vi "Periodic Tasks.vi"(8 "error in":errorcluster) -> ()   [LabVIEW 2015]
doc: "This VI runs in parallel to other tasks. It can contain as many user-defined periodic loops as you need. These can carry out PID or other sorts of timed response."
uses:
  <vilib>/Rock Robotics/WPI/CAN/TalonSRX/WPI_CANTalonSRX_APIControlMode.ctl
  Robot Global Data.vi
  <vilib>/Rock Robotics/Network Tables/NT Write String.vi
  <vilib>/Rock Robotics/WPI/Utilities/WPI_GetSetVariantRefNum.vi
  <vilib>/Rock Robotics/Network Tables/SD Write Numeric Array.vi
  <vilib>/Rock Robotics/Network Tables/SD Write Boolean Array.vi
panel:
  # "PERIODIC TASKS.VI"
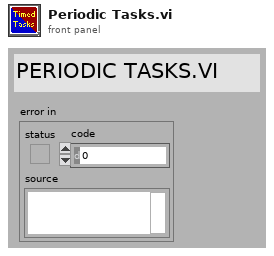
[diagram p1: front panel]
types:
  T1 = typedef "WPI_CANTalonSRX_APIControlMode.ctl" = enum8{"Percent VBus", "Speed", "Position", "Slave", "Unchanged / Invalid", "Voltage Compensation", "Current", "Motion Profile"}
  T2 = typedef "WPI_MotorControlDeviceRef.ctl" = cluster{"DeviceStatus":errorcluster, "Type":T3, "PWM":cluster{"PWM Channel":T4, "DeadBand":T5}, "CAN":cluster{"Device Number":u8, "Control Mode":T6, "Semaphore":T7, "Max Vout":dbl, "TalonSRX Control Mode":T1}, "Invert":bool}
  T3 = typedef "WPI_MotorControlType.ctl" = enum16{"PWM", "CAN", "CANTalonSRX"}
  T4 = typedef "FPGA_DIOPWMChannel.ctl" = enum8{"PWM 0", "PWM 1", "PWM 2", "PWM 3", "PWM 4", "PWM 5", "PWM 6", "PWM 7", "PWM 8", "PWM 9", "PWM MXP 0", "PWM MXP 1", "PWM MXP 2", "PWM MXP 3", "PWM MXP 4", "PWM MXP 5", "PWM MXP 6", "PWM MXP 7", "PWM MXP 8", "PWM MXP 9", "Invalid"}
  T5 = typedef "WPI_PWMDeadband.ctl" = cluster{"Name":string, "maxPositivePwm":i32, "minPositivePwm":i32, "centerPwm":i32, "maxNegativePwm":i32, "minNegativePwm":i32, "angularRange":u16}
  T6 = typedef "WPI_CANJaguar_ControlMode.ctl" = enum8{"Percent VBus", "Current", "Speed", "Position", "Voltage"}
  T7 = typedef "Semaphore RefNum" = refnum<k1>
  T8 = typedef "WPI_JoystickDevRef.ctl" = cluster{"Device":T9}
  T9 = typedef "WPI_JoystickDeviceEnum.ctl" = enum16{"USB 0", "USB 1", "USB 2", "USB 3", "USB 4", "USB 5"}
  T10 = typedef "WPI_ServoDeviceRef.ctl" = cluster{"DeviceStatus":errorcluster, "PWM Channel":T4, "DeadBand":T5}
  T11 = typedef "WPI_PotentiometerDevRef.ctl" = cluster{"DevStatus":errorcluster, "Analog Channel":T12, "Invert Output":bool}
  T12 = typedef "FPGA_AIChannel.ctl" = enum8{"AI 0", "AI 1", "AI 2", "AI 3", "AI MXP 0", "AI MXP 1", "AI MXP 2", "AI MXP 3", "Invalid"}
  T13 = typedef "WPI_SwitchDevRef.ctl" = cluster{"DevStatus":errorcluster, "DIO Channel":T14, "CntIndex":T15, "Normally Closed":bool}
  T14 = typedef "FPGA_DIOChannel.ctl" = enum8{"DIO 0", "DIO 1", "DIO 2", "DIO 3", "DIO 4", "DIO 5", "DIO 6", "DIO 7", "DIO 8", "DIO 9", "DIO MXP 0", "DIO MXP 1", "DIO MXP 2", "DIO MXP 3", "DIO MXP 4", "DIO MXP 5", "DIO MXP 6", "DIO MXP 7", "DIO MXP 8", "DIO MXP 9", "DIO MXP 10", "DIO MXP 11", "DIO MXP 12", "DIO MXP 13", "DIO MXP 14", "DIO MXP 15", "Invalid"}
  T15 = typedef "FPGA_CounterCtrSystemIndex.ctl" = enum8{"Ctr 0", "Ctr 1", "Ctr 2", "Ctr 3", "Ctr 4", "Ctr 5", "Ctr 6", "Ctr 7", "Invalid"}
  T16 = typedef "WPI_CANTalonSRX_GlobalStatus.ctl" = cluster{"Applied Throttle":dbl, "Module Enabled":bool, "CAN Error":errorcluster, "Closed Loop Error":dbl, "Forward Limit Switch Closed":bool, "Reverse Limit Switch Closed":bool, "Sensor Position":dbl, "Sensor Velocity":dbl, "Current":dbl, "Sticky Fault - Over Temp":bool, "Sticky Fault - Under Voltage":bool, "Sticky Fault - Forward Limit":bool, "Sticky Fault - Reverse Limit":bool, "Sticky Fault - Forward Soft Limit":bool, "Sticky Fault - Reverse Soft Limit":bool, "Brake is Enabled":bool, "Encoder Position":dbl, "Encoder Velocity":dbl, "Encoder Index Count":dbl, "Encoder A Pin State":bool, "Encoder B Pin State":bool, "Encoder Index Pin State":bool, "Analog In":dbl, "Analog In Velocity":dbl, "Temperature (C)":dbl, "Battery Voltage":dbl, "Control 5 Is Supported":bool, "Current Profile Slot Select":dbl, "Pos Div 8":bool, "Vel Div 4":bool, "Pulse Width Position":i32, "Pulse Width Velocity":i32, "Pulse Width Rise To Rise (us)":i32, "Pulse Width Rise To Fall (us)":i32, "Mot Prof Active Is Under Run":bool, "Mot Prof Active Has Under Run":bool, "Mot Prof Active Is Last":bool, "Mot Prof Active Velocity Only":bool, "Mot Prof Active Is Valid":bool, "Mot Prof Buffer Is Full":bool, "Mot Prof Active Profile Slot Select":i32, "Mot Prof NextID":i32, "Mot Prof Count":i32, "Mot Prof Active Velocity":dbl, "Mot Prof Active Position":dbl, "Mot Prof Output Enable":i32}
  T17 = typedef "WPI_AnalogChannelDevRef.ctl" = cluster{"DevStatus":errorcluster, "Analog Channel":T12}
  T18 = typedef "WPI_DigitalOutputDevRef.ctl" = cluster{"DIO Channel":T14, "DevStatus":errorcluster}
  T19 = typedef "WPI_GyroDevRef.ctl" = cluster{"DevStatus":errorcluster, "Analog Channel":T12, "Offset":dbl, "Gain (VoltsPerDegree/Second)":dbl, "Gyro Type":enum16{"Analog", "XRS450"}, "Handle":i32, "SPI Bus":T20, "Device Found":bool, "Sample Rate":dbl, "Calibrate On Open":bool}
  T20 = typedef "spi_bus.ctl" = enum16{"SPI On-Board, CS0", "SPI On-Board, CS1", "SPI On-Board, CS2", "SPI On-Board, CS3", "SPI MXP", "Invalid"}
  T21 = typedef "WPI_I2CDevRef.ctl" = cluster{"DevStatus":errorcluster, "Device Address":u8, "Handle":i32, "I2C Bus":T22}
  T22 = typedef "i2c_bus.ctl" = enum16{"I2C On-Board", "I2C MXP", "Invalid"}
  T23 = typedef "WPI_AccelerometerDevRef.ctl" = cluster{"DevStatus":errorcluster, "Scaling":T24, "Analog Channels":T25, "I2C Bus":T22, "SPI Bus":T20, "Accel Range":T26, "ADXL Axes":T27, "Handle":i32, "Device Address":u8, "Accel Type":enum16{"Analog", "ADXL345 I2C", "ADXL345 SPI", "Internal", "ADXL362 SPI"}}
  T24 = typedef "WPI_AccelerometerScaling.ctl" = cluster{"Gain (VoltsPerG)":dbl, "Center Voltage":dbl}
  T25 = typedef "WPI_AccelerometerAnalogChannels.ctl" = cluster{"X-Axis":T12, "Y-Axis":T12, "Z-Axis":T12}
  T26 = typedef "ADXL345 Range.ctl" = u8
  T27 = typedef "WPI_AccelerometerADXL345 Axes.ctl" = cluster{"X-Axis":bool, "Y-Axis":bool, "Z-Axis":bool}
  T28 = cluster{"X-Axis":dbl, "Y-Axis":dbl, "Z-Axis":dbl}
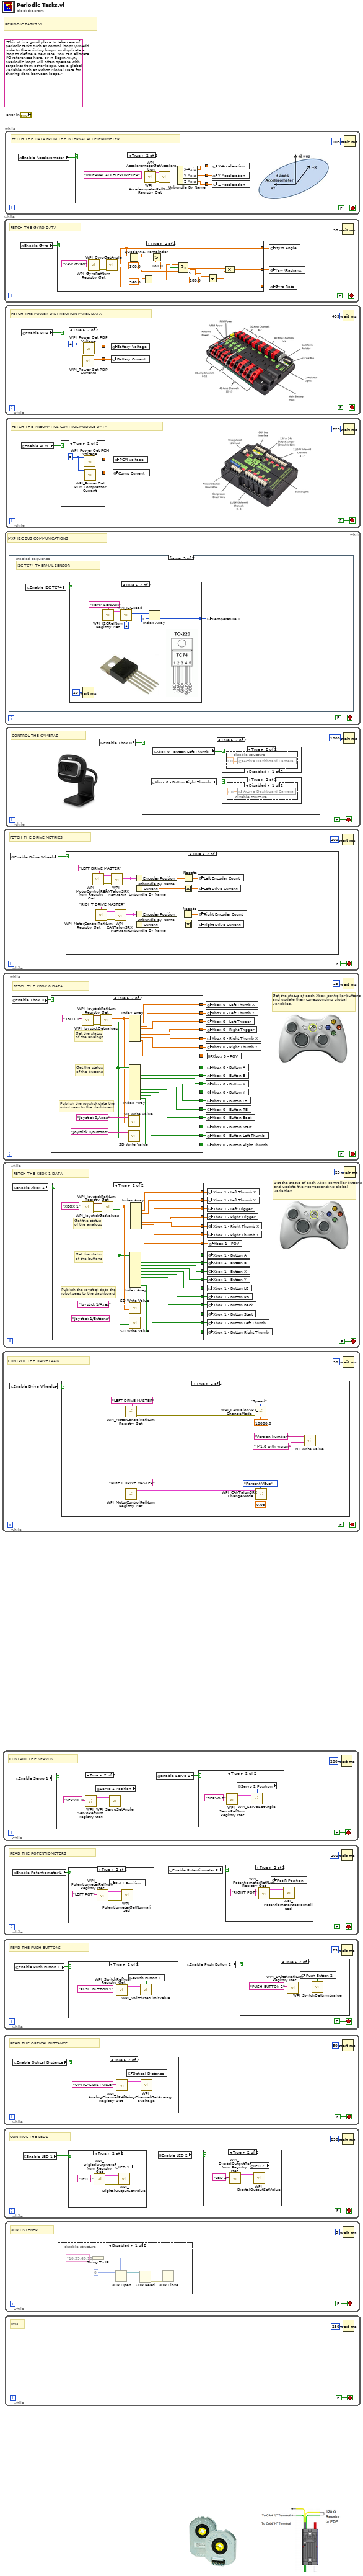
[diagram p0: block diagram]
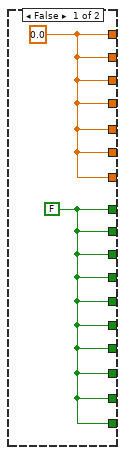
[diagram p12: hidden frame]
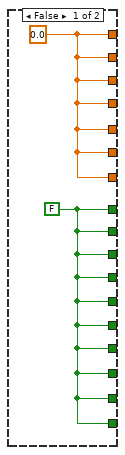
[diagram p13: hidden frame]
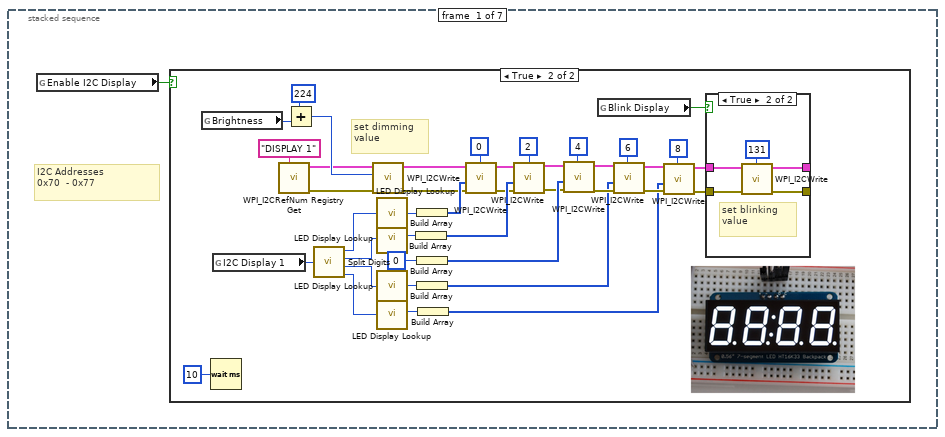
[diagram p14: hidden frame]
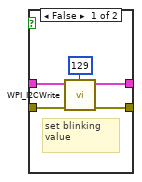
[diagram p16: hidden frame]
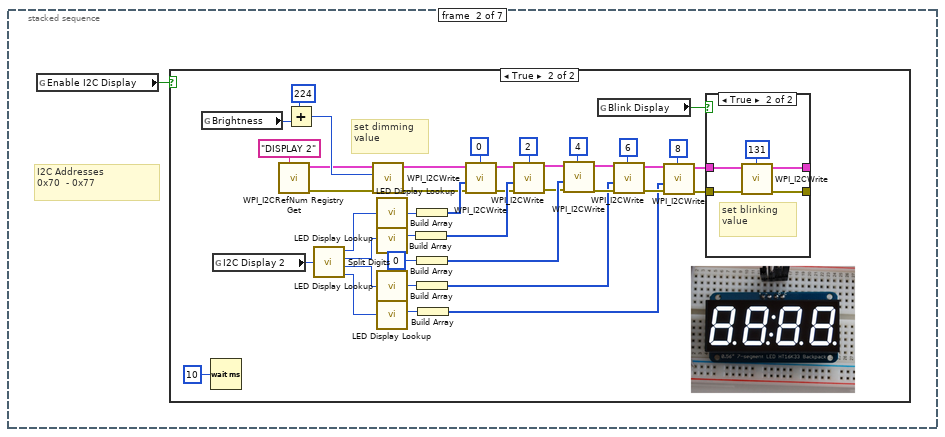
[diagram p17: hidden frame]
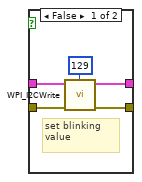
[diagram p19: hidden frame]
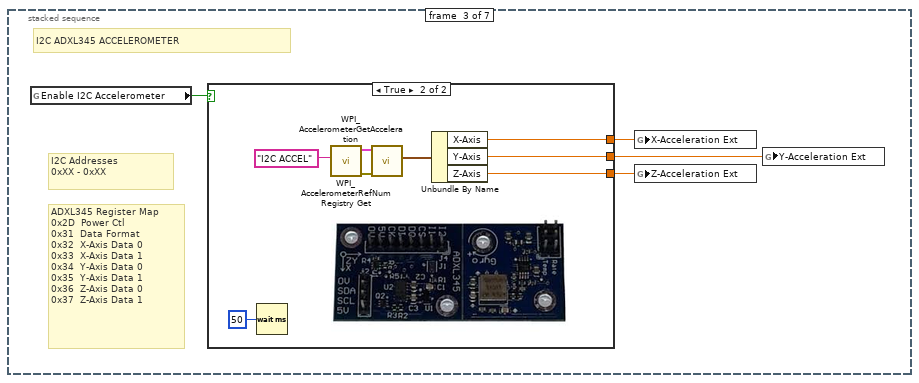
[diagram p20: hidden frame]
diagram:
  (unwired) "This VI is a good place to take care of periodic tasks such as control loops.\n\nAdd code to the existing loops, or duplicate a loop to define a new rate. You can allocate I/O references here, or in Begin.vi.\n\nPeriodic loops will often operate with setpoints from other loops. Use a global variable such as Robot Global Data for sharing data between loops."
  # "PERIODIC TASKS.VI"
  n1 = while {
    stop <- FALSE stop-if-true
    # "CONTROL THE DRIVETRAIN"
    n2 = global read "Robot Global Data.vi" "Enable Drive Wheels"() -> (w1:bool)
    n3 = case shown="True" w1 {
      frame False {
      }
      frame True {
        n4 = call <vilib>:"WPI_MotorControlRefNum Registry Get.vi"("refnum name"="LEFT DRIVE MASTER") -> ("error out"=w13:errorcluster, "MotorControlDevRef"=w14:T2)  [unwired: 9 in]
        n5 = call <vilib>:"WPI_MotorControlRefNum Registry Get.vi"("refnum name"="RIGHT DRIVE MASTER") -> ("error out"=w4:errorcluster, "MotorControlDevRef"=w5:T2)  [unwired: 9 in]
        n6 = call <vilib>:"WPI_CANTalonSRX_ChangeMode.vi"("error in (no error)"=w13, "Output"=10000.0, "Control Mode"=WPI_CANTalonSRX_APIControlMode."Speed", "CAN Talon SRX Ref"=w14) -> ()  [unwired: 6 in, 2 out]
        n7 = call <vilib>:"WPI_CANTalonSRX_ChangeMode.vi"("error in (no error)"=w4, "Output"=0.09, "Control Mode"=WPI_CANTalonSRX_APIControlMode."Percent VBus", "CAN Talon SRX Ref"=w5) -> ()  [unwired: 6 in, 2 out]
        n8 = call-poly <vilib>:"NT Write Value.vi"("String"=" M1.0 with vision", "Name"="Version Number") -> ()  [unwired: 9 in, 1 out]
      }
    }
    n9 = Wait (ms)(milliseconds to wait=u32 50) -> ()  [unwired: 1 out]
  }
  n10 = while {
    stop <- FALSE stop-if-true
    # "Get the status of each Xbox controller buttons and update their corresponding global variables."
    # "FETCH THE XBOX 0 DATA"
    n11 = global read "Robot Global Data.vi" "Enable Xbox 0"() -> (w35:bool)
    n12 = case shown="True" w35 {
      tunnel: [w36 w61] -> w34
      tunnel: [w36 w60] -> w33
      tunnel: [w36 w59] -> w32
      tunnel: [w37 w58] -> w31
      tunnel: [w37 w57] -> w30
      tunnel: [w37 w56] -> w29
      tunnel: [w37 w55] -> w28
      tunnel: [w37 w54] -> w27
      tunnel: [w37 w53] -> w26
      tunnel: [w37 w52] -> w25
      tunnel: [w37 w51] -> w24
      tunnel: [w37 w50] -> w23
      tunnel: [w37 w49] -> w22
      tunnel: [w36 w48] -> w21
      tunnel: [w36 w47] -> w20
      tunnel: [w36 w46] -> w19
      tunnel: [w36 w45] -> w18
      frame False {
        w36 = 0.0 ("upper limit")
        w37 = FALSE
      }
      frame True {
        # "Publish the joystick data the\nrobot sees to the dashboard"
        # "Get the status\nof the analogs"
        # "Get the status\nof the buttons"
        n13 = call <vilib>:"WPI_JoystickRefNum Registry Get.vi"("refnum name"="XBOX 0") -> ("error out"=w38:errorcluster, "JoystickDevRef"=w39:T8)  [unwired: 9 in]
        n14 = call <vilib>:"WPI_JoystickGetValues.vi"("error in (no error)"=w38, "JoystickDevRef"=w39) -> ("Buttons"=w42:bool[], "Axes"=w41:dbl[])  [unwired: 5 in, 3 out]
        n15 = call-poly <vilib>:"SD Write Value.vi"("Numeric Array"=w41, "Name"="Joystick 0/Axes") -> ()  [unwired: 8 in, 2 out]
        n16 = call-poly <vilib>:"SD Write Value.vi"("Boolean Array"=w42, "Name"="Joystick 0/Buttons") -> ()  [unwired: 8 in, 2 out]
        n17 = Index Array(array=w42) -> (element #1=w58:bool, element #2=w57:bool, element #3=w56:bool, element #4=w55:bool, element #5=w54:bool, element #6=w53:bool, element #7=w52:bool, element #8=w51:bool, element #9=w50:bool, element #10=w49:bool)  [unwired: 10 in]
        n18 = Index Array(array=w41) -> (element #1=w61:dbl, element #2=w60:dbl, element #3=w59:dbl, element #4=w48:dbl, element #5=w47:dbl, element #6=w46:dbl, element #7=w45:dbl)  [unwired: 7 in]
      }
    }
    n19 = global write "Robot Global Data.vi" "Xbox 0 - Left Thumb X"(w34) -> ()
    n20 = global write "Robot Global Data.vi" "Xbox 0 - Left Thumb Y"(w33) -> ()
    n21 = global write "Robot Global Data.vi" "Xbox 0 - Left Trigger"(w32) -> ()
    n22 = global write "Robot Global Data.vi" "Xbox 0 - Right Trigger"(w21) -> ()
    n23 = global write "Robot Global Data.vi" "Xbox 0 - Right Thumb X"(w20) -> ()
    n24 = global write "Robot Global Data.vi" "Xbox 0 - Right Thumb Y"(w19) -> ()
    n25 = global write "Robot Global Data.vi" "Xbox 0 - Button A"(w31) -> ()
    n26 = global write "Robot Global Data.vi" "Xbox 0 - Button B"(w30) -> ()
    n27 = global write "Robot Global Data.vi" "Xbox 0 - Button X"(w29) -> ()
    n28 = global write "Robot Global Data.vi" "Xbox 0 - Button Y"(w28) -> ()
    n29 = global write "Robot Global Data.vi" "Xbox 0 - Button LB"(w27) -> ()
    n30 = global write "Robot Global Data.vi" "Xbox 0 - Button RB"(w26) -> ()
    n31 = global write "Robot Global Data.vi" "Xbox 0 - Button Back"(w25) -> ()
    n32 = global write "Robot Global Data.vi" "Xbox 0 - Button Start"(w24) -> ()
    n33 = global write "Robot Global Data.vi" "Xbox 0 - Button Left Thumb"(w23) -> ()
    n34 = global write "Robot Global Data.vi" "Xbox 0 - Button Right Thumb"(w22) -> ()
    n35 = global write "Robot Global Data.vi" "Xbox 0 - POV"(w18) -> ()
    n36 = Wait (ms)(milliseconds to wait=u32 25) -> ()  [unwired: 1 out]
  }
  n37 = while {
    stop <- FALSE stop-if-true
    # "Get the status of each Xbox controller buttons and update their corresponding global variables."
    # "FETCH THE XBOX 1 DATA"
    n38 = global read "Robot Global Data.vi" "Enable Xbox 1"() -> (w81:bool)
    n39 = case shown="True" w81 {
      tunnel: [w82 w107] -> w80
      tunnel: [w82 w106] -> w79
      tunnel: [w82 w105] -> w78
      tunnel: [w83 w104] -> w77
      tunnel: [w83 w103] -> w76
      tunnel: [w83 w102] -> w75
      tunnel: [w83 w101] -> w74
      tunnel: [w83 w100] -> w73
      tunnel: [w83 w99] -> w72
      tunnel: [w83 w98] -> w71
      tunnel: [w83 w97] -> w70
      tunnel: [w83 w96] -> w69
      tunnel: [w83 w95] -> w68
      tunnel: [w82 w94] -> w67
      tunnel: [w82 w93] -> w66
      tunnel: [w82 w92] -> w65
      tunnel: [w82 w91] -> w64
      frame False {
        w82 = 0.0 ("upper limit")
        w83 = FALSE
      }
      frame True {
        # "Publish the joystick data the\nrobot sees to the dashboard"
        # "Get the status\nof the analogs"
        # "Get the status\nof the buttons"
        n40 = call <vilib>:"WPI_JoystickRefNum Registry Get.vi"("refnum name"="XBOX 1") -> ("error out"=w84:errorcluster, "JoystickDevRef"=w85:T8)  [unwired: 9 in]
        n41 = call <vilib>:"WPI_JoystickGetValues.vi"("error in (no error)"=w84, "JoystickDevRef"=w85) -> ("Buttons"=w87:bool[], "Axes"=w88:dbl[])  [unwired: 5 in, 3 out]
        n42 = call-poly <vilib>:"SD Write Value.vi"("Numeric Array"=w88, "Name"="Joystick 1/Axes") -> ()  [unwired: 8 in, 2 out]
        n43 = call-poly <vilib>:"SD Write Value.vi"("Boolean Array"=w87, "Name"="Joystick 1/Buttons") -> ()  [unwired: 8 in, 2 out]
        n44 = Index Array(array=w87) -> (element #1=w104:bool, element #2=w103:bool, element #3=w102:bool, element #4=w101:bool, element #5=w100:bool, element #6=w99:bool, element #7=w98:bool, element #8=w97:bool, element #9=w96:bool, element #10=w95:bool)  [unwired: 10 in]
        n45 = Index Array(array=w88) -> (element #1=w107:dbl, element #2=w106:dbl, element #3=w105:dbl, element #4=w94:dbl, element #5=w93:dbl, element #6=w92:dbl, element #7=w91:dbl)  [unwired: 7 in]
      }
    }
    n46 = global write "Robot Global Data.vi" "Xbox 1 - Left Thumb X"(w80) -> ()
    n47 = global write "Robot Global Data.vi" "Xbox 1 - Left Thumb Y"(w79) -> ()
    n48 = global write "Robot Global Data.vi" "Xbox 1 - Left Trigger"(w78) -> ()
    n49 = global write "Robot Global Data.vi" "Xbox 1 - Right Trigger"(w67) -> ()
    n50 = global write "Robot Global Data.vi" "Xbox 1 - Right Thumb X"(w66) -> ()
    n51 = global write "Robot Global Data.vi" "Xbox 1 - Right Thumb Y"(w65) -> ()
    n52 = global write "Robot Global Data.vi" "Xbox 1 - Button A"(w77) -> ()
    n53 = global write "Robot Global Data.vi" "Xbox 1 - Button B"(w76) -> ()
    n54 = global write "Robot Global Data.vi" "Xbox 1 - Button X"(w75) -> ()
    n55 = global write "Robot Global Data.vi" "Xbox 1 - Button Y"(w74) -> ()
    n56 = global write "Robot Global Data.vi" "Xbox 1 - Button LB"(w73) -> ()
    n57 = global write "Robot Global Data.vi" "Xbox 1 - Button RB"(w72) -> ()
    n58 = global write "Robot Global Data.vi" "Xbox 1 - Button Back"(w71) -> ()
    n59 = global write "Robot Global Data.vi" "Xbox 1 - Button Start"(w70) -> ()
    n60 = global write "Robot Global Data.vi" "Xbox 1 - Button Left Thumb"(w69) -> ()
    n61 = global write "Robot Global Data.vi" "Xbox 1 - Button Right Thumb"(w68) -> ()
    n62 = global write "Robot Global Data.vi" "Xbox 1 - POV"(w64) -> ()
    n63 = Wait (ms)(milliseconds to wait=u32 25) -> ()  [unwired: 1 out]
  }
  n64 = while {
    stop <- FALSE stop-if-true
    # "CONTROL THE SERVOS"
    n65 = global read "Robot Global Data.vi" "Enable Servo 1"() -> (w109:bool)
    n66 = case shown="True" w109 {
      frame False {
      }
      frame True {
        n67 = call <vilib>:"WPI_ServoRefNum Registry Get.vi"("refnum name"="SERVO 1") -> ("error out"=w118:errorcluster, "ServoDeviceRef"=w117:T10)  [unwired: 9 in]
        n68 = global read "Robot Global Data.vi" "Servo 1 Position"() -> (w116:i32)
        n69 = call <vilib>:"WPI_ServoSetAngle.vi"("error in (no error)"=w118, "Angle"=w116, "ServoDeviceRef"=w117) -> ()  [unwired: 7 in, 2 out]
      }
    }
    n70 = global read "Robot Global Data.vi" "Enable Servo 1"() -> (w108:bool)
    n71 = case shown="True" w108 {
      frame False {
      }
      frame True {
        n72 = call <vilib>:"WPI_ServoRefNum Registry Get.vi"("refnum name"="SERVO 2") -> ("error out"=w114:errorcluster, "ServoDeviceRef"=w113:T10)  [unwired: 9 in]
        n73 = global read "Robot Global Data.vi" "Servo 2 Position"() -> (w112:i32)
        n74 = call <vilib>:"WPI_ServoSetAngle.vi"("error in (no error)"=w114, "Angle"=w112, "ServoDeviceRef"=w113) -> ()  [unwired: 7 in, 2 out]
      }
    }
    n75 = Wait (ms)(milliseconds to wait=u32 200) -> ()  [unwired: 1 out]
  }
  n76 = while {
    stop <- FALSE stop-if-true
    # "READ THE POTENTIOMETERS"
    n77 = global read "Robot Global Data.vi" "Enable Potentiometer L"() -> (w121:bool)
    n78 = case shown="True" w121 {
      frame False {
      }
      frame True {
        n79 = call <vilib>:"WPI_PotentiometerRefNum Registry Get.vi"("refnum name"="LEFT POT") -> ("error out"=w130:errorcluster, "PotDevRef"=w129:T11)  [unwired: 9 in]
        n80 = call <vilib>:"WPI_PotentiometerGetNormalized.vi"("error in"=w130, "PotDevRef"=w129) -> ("Normalized Value"=w128:dbl)  [unwired: 7 in, 2 out]
        n81 = global write "Robot Global Data.vi" "Pot L Position"(w128) -> ()
      }
    }
    n82 = global read "Robot Global Data.vi" "Enable Potentiometer R"() -> (w120:bool)
    n83 = case shown="True" w120 {
      frame False {
      }
      frame True {
        n84 = call <vilib>:"WPI_PotentiometerRefNum Registry Get.vi"("refnum name"="RIGHT POT") -> ("error out"=w126:errorcluster, "PotDevRef"=w125:T11)  [unwired: 9 in]
        n85 = call <vilib>:"WPI_PotentiometerGetNormalized.vi"("error in"=w126, "PotDevRef"=w125) -> ("Normalized Value"=w124:dbl)  [unwired: 7 in, 2 out]
        n86 = global write "Robot Global Data.vi" "Pot R Position"(w124) -> ()
      }
    }
    n87 = Wait (ms)(milliseconds to wait=u32 200) -> ()  [unwired: 1 out]
  }
  n88 = while {
    stop <- FALSE stop-if-true
    # "READ THE PUSH BUTTONS"
    n89 = global read "Robot Global Data.vi" "Enable Push Button 1"() -> (w133:bool)
    n90 = case shown="True" w133 {
      frame False {
      }
      frame True {
        n91 = call <vilib>:"WPI_SwitchRefNum Registry Get.vi"("refnum name"="PUSH BUTTON 1") -> ("error out"=w142:errorcluster, "SwitchDevRef"=w141:T13)  [unwired: 9 in]
        n92 = call <vilib>:"WPI_SwitchGetLimitValue.vi"("error in (no error)"=w142, "SwitchDevRef"=w141) -> ("Switch Pressed"=w140:bool)  [unwired: 7 in, 2 out]
        n93 = global write "Robot Global Data.vi" "Push Button 1"(w140) -> ()
      }
    }
    n94 = global read "Robot Global Data.vi" "Enable Push Button 2"() -> (w132:bool)
    n95 = case shown="True" w132 {
      frame False {
      }
      frame True {
        n96 = call <vilib>:"WPI_SwitchRefNum Registry Get.vi"("refnum name"="PUSH BUTTON 2") -> ("error out"=w138:errorcluster, "SwitchDevRef"=w137:T13)  [unwired: 9 in]
        n97 = call <vilib>:"WPI_SwitchGetLimitValue.vi"("error in (no error)"=w138, "SwitchDevRef"=w137) -> ("Switch Pressed"=w136:bool)  [unwired: 7 in, 2 out]
        n98 = global write "Robot Global Data.vi" "Push Button 2"(w136) -> ()
      }
    }
    n99 = Wait (ms)(milliseconds to wait=u32 25) -> ()  [unwired: 1 out]
  }
  n100 = while {
    stop <- FALSE stop-if-true
    # "FETCH THE DRIVE METRICS"
    n101 = global read "Robot Global Data.vi" "Enable Drive Wheels"() -> (w144:bool)
    n102 = case shown="True" w144 {
      frame False {
      }
      frame True {
        n103 = call <vilib>:"WPI_MotorControlRefNum Registry Get.vi"("refnum name"="LEFT DRIVE MASTER") -> ("error out"=w160:errorcluster, "MotorControlDevRef"=w161:T2)  [unwired: 9 in]
        n104 = call <vilib>:"WPI_MotorControlRefNum Registry Get.vi"("refnum name"="RIGHT DRIVE MASTER") -> ("error out"=w157:errorcluster, "MotorControlDevRef"=w158:T2)  [unwired: 9 in]
        n105 = call <vilib>:"WPI_CANTalonSRX_GetStatus.vi"("error in (no error)"=w160, "CAN Talon SRX Ref"=w161) -> ("Talon SRX Status"=w151:T16)  [unwired: 7 in, 2 out]
        n106 = call <vilib>:"WPI_CANTalonSRX_GetStatus.vi"("error in (no error)"=w157, "CAN Talon SRX Ref"=w158) -> ("Talon SRX Status"=w156:T16)  [unwired: 7 in, 2 out]
        n107 = Unbundle By Name(w151) -> ("Encoder Position"=w149:dbl)
        n108 = Unbundle By Name(w151) -> ("Current"=w153:dbl)
        n109 = Unbundle By Name(w156) -> ("Encoder Position"=w148:dbl)
        n110 = Unbundle By Name(w156) -> ("Current"=w155:dbl)
        n111 = Negate(x=w148) -> (-x=w147:dbl)
        n112 = Absolute Value(x=w153) -> (abs(x)=w152:dbl)
        n113 = Absolute Value(x=w155) -> (abs(x)=w154:dbl)
        n114 = Negate(x=w149) -> (-x=w150:dbl)
        n115 = global write "Robot Global Data.vi" "Left Encoder Count"(w150) -> ()
        n116 = global write "Robot Global Data.vi" "Left Drive Current"(w152) -> ()
        n117 = global write "Robot Global Data.vi" "Right Encoder Count"(w147) -> ()
        n118 = global write "Robot Global Data.vi" "Right Drive Current"(w154) -> ()
      }
    }
    n119 = Wait (ms)(milliseconds to wait=u32 200) -> ()  [unwired: 1 out]
  }
  n120 = while {
    stop <- FALSE stop-if-true
    # "READ THE OPTICAL DISTANCE"
    n121 = global read "Robot Global Data.vi" "Enable Optical Distance"() -> (w163:bool)
    n122 = case shown="True" w163 {
      frame False {
      }
      frame True {
        n123 = call <vilib>:"WPI_AnalogChannelRefNum Registry Get.vi"("refnum name"="OPTICAL DISTANCE") -> ("error out"=w168:errorcluster, "AIDeviceRef"=w167:T17)  [unwired: 9 in]
        n124 = call <vilib>:"WPI_AnalogChannelGetAverageVoltage.vi"("error in (no error)"=w168, "AIDeviceRef"=w167) -> ("Voltage"=w166:dbl)  [unwired: 7 in, 2 out]
        n125 = global write "Robot Global Data.vi" "Optical Distance"(w166) -> ()
      }
    }
    n126 = Wait (ms)(milliseconds to wait=u32 50) -> ()  [unwired: 1 out]
  }
  n127 = while {
    stop <- FALSE stop-if-true
    # "CONTROL THE LEDS"
    n128 = global read "Robot Global Data.vi" "Enable LED 1"() -> (w171:bool)
    n129 = case shown="True" w171 {
      frame False {
      }
      frame True {
        n130 = call <vilib>:"WPI_DigitalOutputRefNum Registry Get.vi"("refnum name"="LED 1") -> ("error out"=w180:errorcluster, "DigitalOutputDevRef"=w179:T18)  [unwired: 9 in]
        n131 = global read "Robot Global Data.vi" "LED 1"() -> (w178:bool)
        n132 = call <vilib>:"WPI_DigitalOutputSetValue.vi"("error in (no error)"=w180, "Value"=w178, "DigitalOutputDevRef"=w179) -> ()  [unwired: 7 in, 2 out]
      }
    }
    n133 = global read "Robot Global Data.vi" "Enable LED 2"() -> (w170:bool)
    n134 = case shown="True" w170 {
      frame False {
      }
      frame True {
        n135 = call <vilib>:"WPI_DigitalOutputRefNum Registry Get.vi"("refnum name"="LED 2") -> ("error out"=w176:errorcluster, "DigitalOutputDevRef"=w175:T18)  [unwired: 9 in]
        n136 = global read "Robot Global Data.vi" "LED 2"() -> (w174:bool)
        n137 = call <vilib>:"WPI_DigitalOutputSetValue.vi"("error in (no error)"=w176, "Value"=w174, "DigitalOutputDevRef"=w175) -> ()  [unwired: 7 in, 2 out]
      }
    }
    n138 = Wait (ms)(milliseconds to wait=u32 250) -> ()  [unwired: 1 out]
  }
  n139 = while {
    stop <- FALSE stop-if-true
    # "FETCH THE GYRO DATA"
    n140 = global read "Robot Global Data.vi" "Enable Gyro"() -> (w185:bool)
    n141 = case shown="True" w185 {
      tunnel: [w188 w200] -> w183
      tunnel: [w188 w204] -> w184
      tunnel: [w188 w189] -> w182
      frame False {
        w188 = 0.0
      }
      frame True {
        n142 = call <vilib>:"WPI_GyroRefNum Registry Get.vi"("refnum name"="YAW GYRO") -> ("error out"=w201:errorcluster, "GyroDevRef"=w202:T19)  [unwired: 9 in]
        n143 = call <vilib>:"WPI_GyroGetAngle.vi"("error in"=w201, "GyroDevRef"=w202) -> ("Angular Rate"=w204:dbl, "Angle"=w200:dbl)  [unwired: 5 in, 3 out]
        n144 = Quotient & Remainder(x=w200, y=360.0) -> (x-y*floor(x/y)=w194:dbl)  [unwired: 1 out]
        n145 = Subtract(x=w194, y=360.0) -> (x-y=w195:dbl)
        n146 = Greater?(x=w194, y=180.0) -> (0:w196:bool)
        n147 = Select(t=w195, s=w196, f=w194) -> (s? t:f=w191:dbl)
        n148 = Divide(x=3.141592653589793, y=180.0) -> (x/y=w190:dbl)
        n149 = Compound Arithmetic op=MULTIPLY(w191, w190) -> (w189:dbl)
      }
    }
    n150 = global write "Robot Global Data.vi" "Gyro Angle"(w183) -> ()
    n151 = global write "Robot Global Data.vi" "Yaw (Radians)"(w182) -> ()
    n152 = global write "Robot Global Data.vi" "Gyro Rate"(w184) -> ()
    n153 = Wait (ms)(milliseconds to wait=u32 97) -> ()  [unwired: 1 out]
  }
  n154 = while {
    stop <- FALSE stop-if-true
    # "MXP I2C BUS COMMUNICATIONS"
    n155 = stacked-sequence {
      frame #0 {
        # "I2C Addresses\n0x70  - 0x77"
        n156 = global read "Robot Global Data.vi" "Enable I2C Display"() -> (w206:bool)
        n157 = case shown="True" w206 {
          frame False {
          }
          frame True {
            # "set dimming value"
            n158 = global read "Robot Global Data.vi" "Brightness"() -> (w223:u8)
            n159 = Wait (ms)(milliseconds to wait=u32 10) -> ()  [unwired: 1 out]
            n160 = global read "Robot Global Data.vi" "I2C Display 1"() -> (w221:u16)
            n161 = call <vilib>:"WPI_I2CRefNum Registry Get.vi"("refnum name"="DISPLAY 1") -> ("error out"=w208:errorcluster, "I2CDevRef"=w209:T21)  [unwired: 9 in]
            n162 = Add(x=u8 224 ("I2CRegister"), y=w223) -> (x+y=w222:u8)
            n163 = call "Split Digits.vi"("Input"=w221) -> ("Digit 4"=w213:u16, "Digit 3"=w214:u16, "Digit 2"=w215:u16, "Digit 1"=w216:u16)
            n164 = call <vilib>:"WPI_I2CWrite.vi"("error in (no error)"=w208, "I2CRegister"=w222, "I2CDevRef"=w209) -> ("error out"=w211:errorcluster, "I2CDevRef"=w212:T21)  [unwired: 7 in]
            n165 = call "LED Display Lookup.vi"("Input"=w213) -> ("Output"=w228:u8)
            n166 = call "LED Display Lookup.vi"("Input"=w214) -> ("Output"=w218:u8)
            n167 = call "LED Display Lookup.vi"("Input"=w215) -> ("Output"=w219:u8)
            n168 = call "LED Display Lookup.vi"("Input"=w216) -> ("Output"=w220:u8)
            n169 = Build Array(w218) -> (w243:u8[])
            n170 = Build Array(w228) -> (w245:u8[])
            n171 = Build Array(u8 0 ("Data To Send")) -> (w239:u8[])
            n172 = Build Array(w219) -> (w232:u8[])
            n173 = Build Array(w220) -> (w229:u8[])
            n174 = call <vilib>:"WPI_I2CWrite.vi"("error in (no error)"=w211, "I2CDataToSend"=w245, "I2CRegister"=u8 0 ("Data To Send"), "I2CDevRef"=w212) -> ("error out"=w241:errorcluster, "I2CDevRef"=w242:T21)  [unwired: 6 in]
            n175 = call <vilib>:"WPI_I2CWrite.vi"("error in (no error)"=w241, "I2CDataToSend"=w243, "I2CRegister"=u8 2 ("Data To Send"), "I2CDevRef"=w242) -> ("error out"=w237:errorcluster, "I2CDevRef"=w238:T21)  [unwired: 6 in]
            n176 = call <vilib>:"WPI_I2CWrite.vi"("error in (no error)"=w237, "I2CDataToSend"=w239, "I2CRegister"=u8 4 ("Data To Send"), "I2CDevRef"=w238) -> ("error out"=w233:errorcluster, "I2CDevRef"=w234:T21)  [unwired: 6 in]
            n177 = global read "Robot Global Data.vi" "Blink Display"() -> (w225:bool)
            n178 = call <vilib>:"WPI_I2CWrite.vi"("error in (no error)"=w233, "I2CDataToSend"=w232, "I2CRegister"=u8 6 ("Data To Send"), "I2CDevRef"=w234) -> ("error out"=w230:errorcluster, "I2CDevRef"=w231:T21)  [unwired: 6 in]
            n179 = call <vilib>:"WPI_I2CWrite.vi"("error in (no error)"=w230, "I2CDataToSend"=w229, "I2CRegister"=u8 8 ("Data To Send"), "I2CDevRef"=w231) -> ("error out"=w226:errorcluster, "I2CDevRef"=w227:T21)  [unwired: 6 in]
            n180 = case shown="True" w225 {
              tunnel: [w248 w255] -> _
              tunnel: [w247 w254] -> _
              tunnel: w227 -> [w250 w253]
              tunnel: w226 -> [w249 w252]
              frame False {
                # "set blinking value"
                n181 = call <vilib>:"WPI_I2CWrite.vi"("error in (no error)"=w249, "I2CRegister"=u8 129, "I2CDevRef"=w250) -> ("error out"=w247:errorcluster, "I2CDevRef"=w248:T21)  [unwired: 7 in]
              }
              frame True {
                # "set blinking value"
                n182 = call <vilib>:"WPI_I2CWrite.vi"("error in (no error)"=w252, "I2CRegister"=u8 131, "I2CDevRef"=w253) -> ("error out"=w254:errorcluster, "I2CDevRef"=w255:T21)  [unwired: 7 in]
              }
            }
          }
        }
      }
      frame #1 {
        # "I2C Addresses\n0x70  - 0x77"
        n183 = global read "Robot Global Data.vi" "Enable I2C Display"() -> (w257:bool)
        n184 = case shown="True" w257 {
          frame False {
          }
          frame True {
            # "set dimming value"
            n185 = global read "Robot Global Data.vi" "Brightness"() -> (w274:u8)
            n186 = Wait (ms)(milliseconds to wait=u32 10) -> ()  [unwired: 1 out]
            n187 = global read "Robot Global Data.vi" "I2C Display 2"() -> (w272:u16)
            n188 = call <vilib>:"WPI_I2CRefNum Registry Get.vi"("refnum name"="DISPLAY 2") -> ("error out"=w259:errorcluster, "I2CDevRef"=w260:T21)  [unwired: 9 in]
            n189 = Add(x=u8 224 ("I2CRegister"), y=w274) -> (x+y=w273:u8)
            n190 = call "Split Digits.vi"("Input"=w272) -> ("Digit 4"=w264:u16, "Digit 3"=w265:u16, "Digit 2"=w266:u16, "Digit 1"=w267:u16)
            n191 = call <vilib>:"WPI_I2CWrite.vi"("error in (no error)"=w259, "I2CRegister"=w273, "I2CDevRef"=w260) -> ("error out"=w262:errorcluster, "I2CDevRef"=w263:T21)  [unwired: 7 in]
            n192 = call "LED Display Lookup.vi"("Input"=w264) -> ("Output"=w279:u8)
            n193 = call "LED Display Lookup.vi"("Input"=w265) -> ("Output"=w269:u8)
            n194 = call "LED Display Lookup.vi"("Input"=w266) -> ("Output"=w270:u8)
            n195 = call "LED Display Lookup.vi"("Input"=w267) -> ("Output"=w271:u8)
            n196 = Build Array(w269) -> (w294:u8[])
            n197 = Build Array(w279) -> (w296:u8[])
            n198 = Build Array(u8 0 ("Data To Send")) -> (w290:u8[])
            n199 = Build Array(w270) -> (w283:u8[])
            n200 = Build Array(w271) -> (w280:u8[])
            n201 = call <vilib>:"WPI_I2CWrite.vi"("error in (no error)"=w262, "I2CDataToSend"=w296, "I2CRegister"=u8 0 ("Data To Send"), "I2CDevRef"=w263) -> ("error out"=w292:errorcluster, "I2CDevRef"=w293:T21)  [unwired: 6 in]
            n202 = call <vilib>:"WPI_I2CWrite.vi"("error in (no error)"=w292, "I2CDataToSend"=w294, "I2CRegister"=u8 2 ("Data To Send"), "I2CDevRef"=w293) -> ("error out"=w288:errorcluster, "I2CDevRef"=w289:T21)  [unwired: 6 in]
            n203 = call <vilib>:"WPI_I2CWrite.vi"("error in (no error)"=w288, "I2CDataToSend"=w290, "I2CRegister"=u8 4 ("Data To Send"), "I2CDevRef"=w289) -> ("error out"=w284:errorcluster, "I2CDevRef"=w285:T21)  [unwired: 6 in]
            n204 = global read "Robot Global Data.vi" "Blink Display"() -> (w276:bool)
            n205 = call <vilib>:"WPI_I2CWrite.vi"("error in (no error)"=w284, "I2CDataToSend"=w283, "I2CRegister"=u8 6 ("Data To Send"), "I2CDevRef"=w285) -> ("error out"=w281:errorcluster, "I2CDevRef"=w282:T21)  [unwired: 6 in]
            n206 = call <vilib>:"WPI_I2CWrite.vi"("error in (no error)"=w281, "I2CDataToSend"=w280, "I2CRegister"=u8 8 ("Data To Send"), "I2CDevRef"=w282) -> ("error out"=w277:errorcluster, "I2CDevRef"=w278:T21)  [unwired: 6 in]
            n207 = case shown="True" w276 {
              tunnel: [w299 w306] -> _
              tunnel: [w298 w305] -> _
              tunnel: w278 -> [w301 w304]
              tunnel: w277 -> [w300 w303]
              frame False {
                # "set blinking value"
                n208 = call <vilib>:"WPI_I2CWrite.vi"("error in (no error)"=w300, "I2CRegister"=u8 129, "I2CDevRef"=w301) -> ("error out"=w298:errorcluster, "I2CDevRef"=w299:T21)  [unwired: 7 in]
              }
              frame True {
                # "set blinking value"
                n209 = call <vilib>:"WPI_I2CWrite.vi"("error in (no error)"=w303, "I2CRegister"=u8 131, "I2CDevRef"=w304) -> ("error out"=w305:errorcluster, "I2CDevRef"=w306:T21)  [unwired: 7 in]
              }
            }
          }
        }
      }
      frame #2 {
        # "I2C Addresses\n0xXX - 0xXX"
        # "ADXL345 Register Map\n0x2D  Power Ctl\n0x31  Data Format\n0x32  X-Axis Data 0\n0x33  X-Axis Data 1\n0x34  Y-Axis Data 0\n0x35  Y-Axis Data 1\n0x36  Z-Axis Data 0\n0x37  Z-Axis Data 1"
        # "I2C ADXL345 ACCELEROMETER"
        n210 = global read "Robot Global Data.vi" "Enable I2C Accelerometer"() -> (w311:bool)
        n211 = case shown="True" w311 {
          tunnel: [0.0 w321] -> w310
          tunnel: [0.0 w320] -> w309
          tunnel: [0.0 w319] -> w308
          frame False {
          }
          frame True {
            n212 = Wait (ms)(milliseconds to wait=u32 50) -> ()  [unwired: 1 out]
            n213 = call <vilib>:"WPI_AccelerometerRefNum Registry Get.vi"("refnum name"="I2C ACCEL") -> ("error out"=w317:errorcluster, "AccelerometerDevRef"=w316:T23)  [unwired: 9 in]
            n214 = call <vilib>:"WPI_AccelerometerGetAcceleration.vi"("error in"=w317, "AccelerometerDevRef"=w316) -> ("Accelerations"=w322:T28)  [unwired: 7 in, 2 out]
            n215 = Unbundle By Name(w322) -> ("X-Axis"=w321:dbl, "Y-Axis"=w320:dbl, "Z-Axis"=w319:dbl)
          }
        }
        n216 = global write "Robot Global Data.vi" "X-Acceleration Ext"(w310) -> ()
        n217 = global write "Robot Global Data.vi" "Z-Acceleration Ext"(w308) -> ()
        n218 = global write "Robot Global Data.vi" "Y-Acceleration Ext"(w309) -> ()
      }
      frame #3 {
        # "I2C Addresses\n0x29  - 0x29"
        # "I2C RGB SENSOR"
        n219 = global read "Robot Global Data.vi" "Enable RGB Sensor"() -> (w327:bool)
        n220 = case shown="True" w327 {
          tunnel: [u16 0 w345] -> w326
          tunnel: [u16 0 w342] -> w323
          tunnel: [u16 0 w341] -> w324
          tunnel: [u16 0 w338] -> w325
          frame False {
          }
          frame True {
            # "enable register"
            # "control register"
            # "timing register"
            n221 = Wait (ms)(milliseconds to wait=u32 50) -> ()  [unwired: 1 out]
            n222 = call <vilib>:"WPI_I2CRefNum Registry Get.vi"("refnum name"="RGB SENSOR") -> ("error out"=w333:errorcluster, "I2CDevRef"=w334:T21)  [unwired: 9 in]
            n223 = Build Array(u8 0 ("Device Address")) -> (w364:u8[])
            n224 = call <vilib>:"WPI_I2CWrite.vi"("error in (no error)"=w333, "I2CDataToSend"=w364, "I2CRegister"=u8 129, "I2CDevRef"=w334) -> ("error out"=w360:errorcluster, "I2CDevRef"=w361:T21)  [unwired: 6 in]
            n225 = Build Array(u8 0 ("Device Address")) -> (w356:u8[])
            n226 = call <vilib>:"WPI_I2CWrite.vi"("error in (no error)"=w360, "I2CDataToSend"=w356, "I2CRegister"=u8 143, "I2CDevRef"=w361) -> ("error out"=w358:errorcluster, "I2CDevRef"=w359:T21)  [unwired: 6 in]
            n227 = Build Array(u8 3 ("Device Address")) -> (w354:u8[])
            n228 = call <vilib>:"WPI_I2CWrite.vi"("error in (no error)"=w358, "I2CDataToSend"=w354, "I2CRegister"=u8 128, "I2CDevRef"=w359) -> ("error out"=w352:errorcluster, "I2CDevRef"=w353:T21)  [unwired: 6 in]
            n229 = Build Array(u8 148 ("Device Address")) -> (w349:u8[])
            n230 = call <vilib>:"WPI_I2CRead.vi"("error in (no error)"=w352, "I2CBytesToRead"=u8 8, "I2CRegister"=w349, "I2CDevRef"=w353) -> ("Data Out"=w348:u8[])  [unwired: 5 in, 2 out]
            n231 = Index Array(array=w348) -> (element #1=w346:u8, element #2=w347:u8, element #3=w344:u8, element #4=w343:u8, element #5=w340:u8, element #6=w339:u8, element #7=w337:u8, element #8=w336:u8)  [unwired: 8 in]
            n232 = Join Numbers(hi=w347, lo=w346) -> ((hi.lo)=w345:u16)
            n233 = Join Numbers(hi=w343, lo=w344) -> ((hi.lo)=w342:u16)
            n234 = Join Numbers(hi=w339, lo=w340) -> ((hi.lo)=w341:u16)
            n235 = Join Numbers(hi=w336, lo=w337) -> ((hi.lo)=w338:u16)
          }
        }
        n236 = global write "Robot Global Data.vi" "RGB Clear"(w326) -> ()
        n237 = global write "Robot Global Data.vi" "RGB Green"(w324) -> ()
        n238 = global write "Robot Global Data.vi" "RGB Blue"(w325) -> ()
        n239 = global write "Robot Global Data.vi" "RGB Red"(w323) -> ()
      }
      frame #4 {
        # "I2C TC74 THERMAL SENSOR"
        n240 = global read "Robot Global Data.vi" "Enable I2C TC74"() -> (w368:bool)
        n241 = case shown="True" w368 {
          tunnel: [u8 0 w372] -> w367
          frame False {
          }
          frame True {
            n242 = Wait (ms)(milliseconds to wait=u32 20) -> ()  [unwired: 1 out]
            n243 = call <vilib>:"WPI_I2CRefNum Registry Get.vi"("refnum name"="TEMP SENSOR") -> ("error out"=w370:errorcluster, "I2CDevRef"=w371:T21)  [unwired: 9 in]
            n244 = call <vilib>:"WPI_I2CRead.vi"("error in (no error)"=w370, "I2CBytesToRead"=u8 1, "I2CDevRef"=w371) -> ("Data Out"=w376:u8[])  [unwired: 6 in, 2 out]
            n245 = Index Array(array=w376, index=0) -> (element=w372:u8)
          }
        }
        n246 = global write "Robot Global Data.vi" "Temperature 1"(w367) -> ()
      }
      frame #5 {
        # "MCP9808"
        n247 = global read "Robot Global Data.vi" "Enable MCP9808"() -> (w379:bool)
        n248 = case shown="True" w379 {
          tunnel: [0.0 w381] -> w378
          frame False {
          }
          frame True {
            # "power up command"
            n249 = Wait (ms)(milliseconds to wait=u32 25) -> ()  [unwired: 1 out]
            n250 = call <vilib>:"WPI_I2CRefNum Registry Get.vi"("refnum name"="MCP9808") -> ("error out"=w393:errorcluster, "I2CDevRef"=w394:T21)  [unwired: 9 in]
            n251 = Build Array(u8 0 ("Device Address")) -> (w396:u8[])
            n252 = call <vilib>:"WPI_I2CWrite.vi"("error in (no error)"=w393, "I2CDataToSend"=w396, "I2CRegister"=u8 5, "I2CDevRef"=w394) -> ("error out"=w392:errorcluster, "I2CDevRef"=w391:T21)  [unwired: 6 in]
            n253 = call <vilib>:"WPI_I2CRead.vi"("error in (no error)"=w392, "I2CBytesToRead"=u8 2, "I2CDevRef"=w391) -> ("Data Out"=w389:u8[])  [unwired: 6 in, 2 out]
            n254 = Index Array(array=w389, index #1=0 ("index")) -> (element #1=w385:u8, element #2=w386:u8)  [unwired: 1 in]
            n255 = Join Numbers(hi=w386, lo=w385) -> ((hi.lo)=w382:u16)
            n256 = To Double Precision Float(number=w382) -> (double precision float=w383:dbl)
            n257 = Divide(x=w383, y=1000.0) -> (x/y=w381:dbl)
          }
        }
        n258 = global write "Robot Global Data.vi" "Temperature 2"(w378) -> ()
      }
      frame #6 {
        # "IR SEEKER"
        n259 = global read "Robot Global Data.vi" "Enable IR Seeker"() -> (w402:bool)
        n260 = case shown="True" w402 {
          tunnel: [w403 w406] -> w401
          tunnel: [w403 w405] -> w400
          tunnel: [w403 w404] -> w399
          frame False {
            w403 = u8 0
          }
          frame True {
            # "power up command"
            n261 = Wait (ms)(milliseconds to wait=u32 25) -> ()  [unwired: 1 out]
            n262 = call <vilib>:"WPI_I2CRefNum Registry Get.vi"("refnum name"="MCP9808") -> ("error out"=w408:errorcluster, "I2CDevRef"=w409:T21)  [unwired: 9 in]
            n263 = call <vilib>:"WPI_I2CRead.vi"("error in (no error)"=w408, "I2CBytesToRead"=u8 16, "I2CDevRef"=w409) -> ("Data Out"=w411:u8[])  [unwired: 6 in, 2 out]
            n264 = Index Array(array=w411, index #1=0 ("index")) -> (element #1=w406:u8, element #2=w405:u8, element #3=w404:u8)  [unwired: 15 in, 13 out]
          }
        }
        n265 = global write "Robot Global Data.vi" "Seeker Firmware"(w401) -> ()
        n266 = global write "Robot Global Data.vi" "Seeker Manufacturer"(w400) -> ()
        n267 = global write "Robot Global Data.vi" "Seeker ID"(w399) -> ()
      }
    }
  }
  n268 = while {
    stop <- FALSE stop-if-true
    # "UDP LISTENER"
    n269 = disable-structure shown="Disabled" {
      frame Disabled {
        n270 = String To IP(1:"10.39.60.10" ("name")) -> (0:w418:u32)
        n271 = UDP Open(7:w418, 11:u16 0 ("port")) -> (port=w419:refnum<k16>, 0:w420:errorcluster)  [unwired: 3 in, 1 out]
        n272 = UDP Read(connection ID=w419, 8:w420) -> (error out=w421:errorcluster, 3:w422:refnum<k16>)  [unwired: 2 in, 3 out]
        n273 = UDP Close(connection ID=w422, 8:w421) -> ()  [unwired: 2 out]
      }
      frame Enabled {
      }
    }
    n274 = Wait (ms)(milliseconds to wait=u32 5) -> ()  [unwired: 1 out]
  }
  n275 = while {
    stop <- FALSE stop-if-true
    # "FETCH THE DATA FROM THE INTERNAL ACCELEROMETER"
    n276 = global read "Robot Global Data.vi" "Enable Accelerometer"() -> (w426:bool)
    n277 = case shown="True" w426 {
      tunnel: [w429 w435] -> w424
      tunnel: [w429 w434] -> w425
      tunnel: [w429 w433] -> w423
      frame False {
        w429 = 0.0
      }
      frame True {
        n278 = call <vilib>:"WPI_AccelerometerRefNum Registry Get.vi"("refnum name"="INTERNAL ACCELEROMETER") -> ("error out"=w430:errorcluster, "AccelerometerDevRef"=w431:T23)  [unwired: 9 in]
        n279 = call <vilib>:"WPI_AccelerometerGetAcceleration.vi"("error in"=w430, "AccelerometerDevRef"=w431) -> ("Accelerations"=w436:T28)  [unwired: 7 in, 2 out]
        n280 = Unbundle By Name(w436) -> ("X-Axis"=w434:dbl, "Y-Axis"=w435:dbl, "Z-Axis"=w433:dbl)
      }
    }
    n281 = global write "Robot Global Data.vi" "X-Acceleration"(w425) -> ()
    n282 = global write "Robot Global Data.vi" "Y-Acceleration"(w424) -> ()
    n283 = global write "Robot Global Data.vi" "Z-Acceleration"(w423) -> ()
    n284 = Wait (ms)(milliseconds to wait=u32 105) -> ()  [unwired: 1 out]
  }
  n285 = while {
    stop <- FALSE stop-if-true
    # "FETCH THE POWER DISTRIBUTION PANEL DATA"
    n286 = global read "Robot Global Data.vi" "Enable PDP"() -> (w439:bool)
    n287 = case shown="True" w439 {
      tunnel: [w442 w445] -> w438
      tunnel: [w442 w444] -> w437
      frame False {
        w442 = 0.0
      }
      frame True {
        w443 = u8 4 ("Power Distribution Panel (0)")
        n288 = call <vilib>:"WPI_Power Get PDP Currents.vi"("Power Distribution Panel (0)"=w443) -> ("current (A)"=w444:dbl)  [unwired: 12 in, 2 out]
        n289 = call <vilib>:"WPI_Power Get PDP Voltage.vi"("Power Distribution Panel (0)"=w443) -> ("voltage (V)"=w445:dbl)  [unwired: 13 in, 1 out]
      }
    }
    n290 = global write "Robot Global Data.vi" "Battery Voltage"(w438) -> ()
    n291 = global write "Robot Global Data.vi" "Battery Current"(w437) -> ()
    n292 = Wait (ms)(milliseconds to wait=u32 459) -> ()  [unwired: 1 out]
  }
  n293 = while {
    stop <- FALSE stop-if-true
    # "IMU"
    n294 = Wait (ms)(milliseconds to wait=u32 250) -> ()  [unwired: 1 out]
  }
  n295 = while {
    stop <- FALSE stop-if-true
    # "FETCH THE PNEUMATICS CONTROL MODULE DATA"
    n296 = global read "Robot Global Data.vi" "Enable PCM"() -> (w450:bool)
    n297 = case shown="True" w450 {
      tunnel: [w453 w456] -> w449
      tunnel: [w453 w454] -> w448
      frame False {
        w453 = 0.0
      }
      frame True {
        w455 = u8 6 ("Power Distribution Panel (0)")
        n298 = call <vilib>:"WPI_Power Get PCM Voltage.vi"("Pneumatics Control Module (0)"=w455) -> ("Input Voltage"=w456:dbl)  [unwired: 12 in, 2 out]
        n299 = call <vilib>:"WPI_Power Get PCM Compressor Current.vi"("Pneumatics Control Module (0)"=w455) -> ("current (A)"=w454:dbl)  [unwired: 13 in, 1 out]
      }
    }
    n300 = global write "Robot Global Data.vi" "Comp Current"(w448) -> ()
    n301 = global write "Robot Global Data.vi" "PCM Voltage"(w449) -> ()
    n302 = Wait (ms)(milliseconds to wait=u32 223) -> ()  [unwired: 1 out]
  }
  n303 = while {
    stop <- FALSE stop-if-true
    # "CONTROL THE CAMERAS"
    n304 = global read "Robot Global Data.vi" "Enable Xbox 0"() -> (w457:bool)
    n305 = case shown="True" w457 {
      frame False {
      }
      frame True {
        n306 = global read "Robot Global Data.vi" "Xbox 0 - Button Right Thumb"() -> (w460:bool)
        n307 = global read "Robot Global Data.vi" "Xbox 0 - Button Left Thumb"() -> (w461:bool)
        n308 = case shown="True" w461 {
          frame False {
          }
          frame True {
            n309 = disable-structure shown="Disabled" {
              frame Disabled {
                n310 = global write "Robot Global Data.vi" "Active Dashboard Camera"(0.0 ("Active Camera")) -> ()
              }
              frame Enabled {
              }
            }
          }
        }
        n311 = case shown="True" w460 {
          frame False {
          }
          frame True {
            n312 = disable-structure shown="Disabled" {
              frame Disabled {
                n313 = global write "Robot Global Data.vi" "Active Dashboard Camera"(1.0 ("Active Camera")) -> ()
              }
              frame Enabled {
              }
            }
          }
        }
      }
    }
    n314 = Wait (ms)(milliseconds to wait=u32 1000) -> ()  [unwired: 1 out]
  }
